vi "Laser_init.vi"(2 "baud rate (9600)":u32=9600, 3 "Laser Repetition\nFrequency":i32, 4 "VISA resource name":refnum<visa-resource-name>="COM10", 5 "Diode Current\nSetting":dbl) -> (0 "error out":errorcluster, 1 "VISA Refnum out":refnum<visa-resource-name>)   [LabVIEW 2019]
uses:
  <vilib>/Instr/_visa.llb/VISA Configure Serial Port (Instr).vi
panel:
  out "read buffer 4":string
  out "read buffer 3":string
  out "read buffer 2":string
  out "read buffer":string
  out "concatenated string 2":string
  out "Diode Current Setting":string
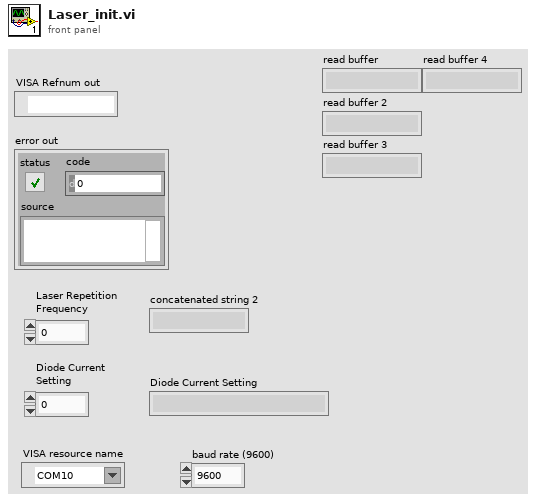
[diagram p1: front panel]
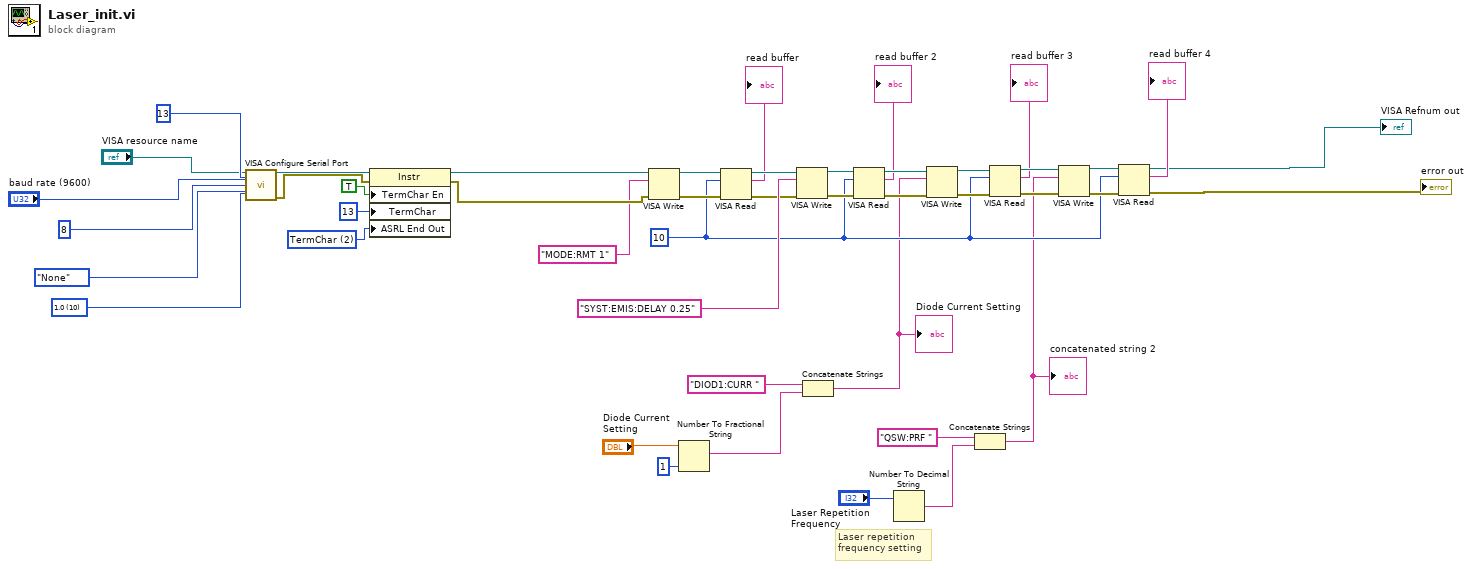
[diagram p0: block diagram]
diagram:
  w19 = u32 10 ("byte count")
  w25 = u16 2 items=["None", "Last Bit", "TermChar", "Break"] ("Serial Settings:End Mode for Writes")
  w29 = u16 10 items=["1.0"=10, "1.5"=15, "2.0"=20] ("stop bits (10: 1 bit)")
  # "Laser repetition\nfrequency setting"
  n1 = call-poly "VISA Configure Serial Port"("VISA resource name"="VISA resource name", "termination char\n(0xA = '\\n' = LF)"=u8 13 ("termination char\n(0xA = '\\n' = LF)"), "baud rate (9600)"="baud rate (9600)", "data bits (8)"=u16 8, "parity (0:none)"=enum16{"None", "Odd", "Even", "Mark", "Space"}."None", "stop bits (10: 1 bit)"=w29) -> ("VISA resource name out"=w22:refnum<visa-resource-name>, "error out"=w30:errorcluster)  [unwired: 8 in]
  n2 = property class="Instr"(reference=w22, error in=w30, "TermChar En"=TRUE ("Message Based Settings:Termination Character Enable"), "TermChar"=u8 13 ("Message Based Settings:Termination Character"), "ASRL End Out"=w25) -> (reference out=w20:refnum<visa-resource-name>, error out=w31:errorcluster)
  n3 = VISA Write(VISA resource name=w20, write buffer="MODE:RMT 1", error in (no error)=w31) -> (VISA resource name out=w35:refnum<visa-resource-name>, error out=w34:errorcluster)  [unwired: 1 out]
  n4 = Number To Fractional String(number="Diode Current\nSetting", precision (6)=i16 1) -> (F-format string=w12:string)  [unwired: 2 in]
  n5 = VISA Read(VISA resource name=w35, byte count=w19, error in (no error)=w34) -> (VISA resource name out=w32:refnum<visa-resource-name>, read buffer=→"read buffer":string, error out=w7:errorcluster)  [unwired: 1 out]
  n6 = VISA Write(VISA resource name=w32, write buffer="SYST:EMIS:DELAY 0.25", error in (no error)=w7) -> (VISA resource name out=w37:refnum<visa-resource-name>, error out=w36:errorcluster)  [unwired: 1 out]
  n7 = Concatenate Strings("DIOD1:CURR " ("string"), w12) -> (w13:string)
  "Diode Current Setting" <- w13
  n8 = VISA Read(VISA resource name=w37, byte count=w19, error in (no error)=w36) -> (VISA resource name out=w40:refnum<visa-resource-name>, read buffer=→"read buffer 2":string, error out=w38:errorcluster)  [unwired: 1 out]
  n9 = Number To Decimal String(number="Laser Repetition\nFrequency") -> (decimal integer string=w15:string)  [unwired: 1 in]
  n10 = VISA Write(VISA resource name=w40, write buffer=w13, error in (no error)=w38) -> (VISA resource name out=w41:refnum<visa-resource-name>, error out=w42:errorcluster)  [unwired: 1 out]
  n11 = Concatenate Strings("QSW:PRF " ("string"), w15) -> (w16:string)
  "concatenated string 2" <- w16
  n12 = VISA Read(VISA resource name=w41, byte count=w19, error in (no error)=w42) -> (VISA resource name out=w39:refnum<visa-resource-name>, read buffer=→"read buffer 3":string, error out=w43:errorcluster)  [unwired: 1 out]
  n13 = VISA Write(VISA resource name=w39, write buffer=w16, error in (no error)=w43) -> (VISA resource name out=w45:refnum<visa-resource-name>, error out=w44:errorcluster)  [unwired: 1 out]
  n14 = VISA Read(VISA resource name=w45, byte count=w19, error in (no error)=w44) -> (VISA resource name out=→"VISA Refnum out":refnum<visa-resource-name>, read buffer=→"read buffer 4":string, error out=→"error out":errorcluster)  [unwired: 1 out]
